vi "1D_Jacobi_eigenvalue_algorithm_v2.vi"() -> ()   [LabVIEW 2020]
uses:
  <vilib>/Analysis/Matrix/Datatypes/RealMatrix.ctl
  <vilib>/Analysis/baseanly.llb/Real A x B.vi
  <vilib>/Analysis/baseanly.llb/Mean (DBL).vi
  <vilib>/Analysis/Matrix/Numeric/Conversions/Array To Matrix - RA2.vi
  <vilib>/Analysis/Matrix/Numeric/Conversions/Matrix To Array - RM.vi
  <vilib>/Analysis/7linalg.llb/Real Eigenvalues and Vectors.vi
  <vilib>/Analysis/Matrix/NI_Matrix.lvlib
  <vilib>/Analysis/NI_AALBase.lvlib
  <vilib>/Analysis/NI_AALPro.lvlib
panel:
  out "New A[k,k]":sgl
  out "[k,k]":i32
  out "after A[k,k]":sgl[][](array[numeric])
  out "before A[k,k]":sgl[][](array[numeric])
  out "Array 3":bool[][](array[boolean])
  out "Numeric":i32
  out "Array 2":i32[](array[numeric])
  out "Array":i32[](array[numeric])
  out "output array":sgl[][](array[numeric])
  out "Real Matrix":T1
  out "percent error":dbl
  out "FPGA Jacobi eigenvalue":sgl[](array[numeric])
  in  "Number of Rotations":i32=100
  out "A":dbl[][](array[numeric])
  out "LabVIEW eigvals":dbl[](array[numeric])
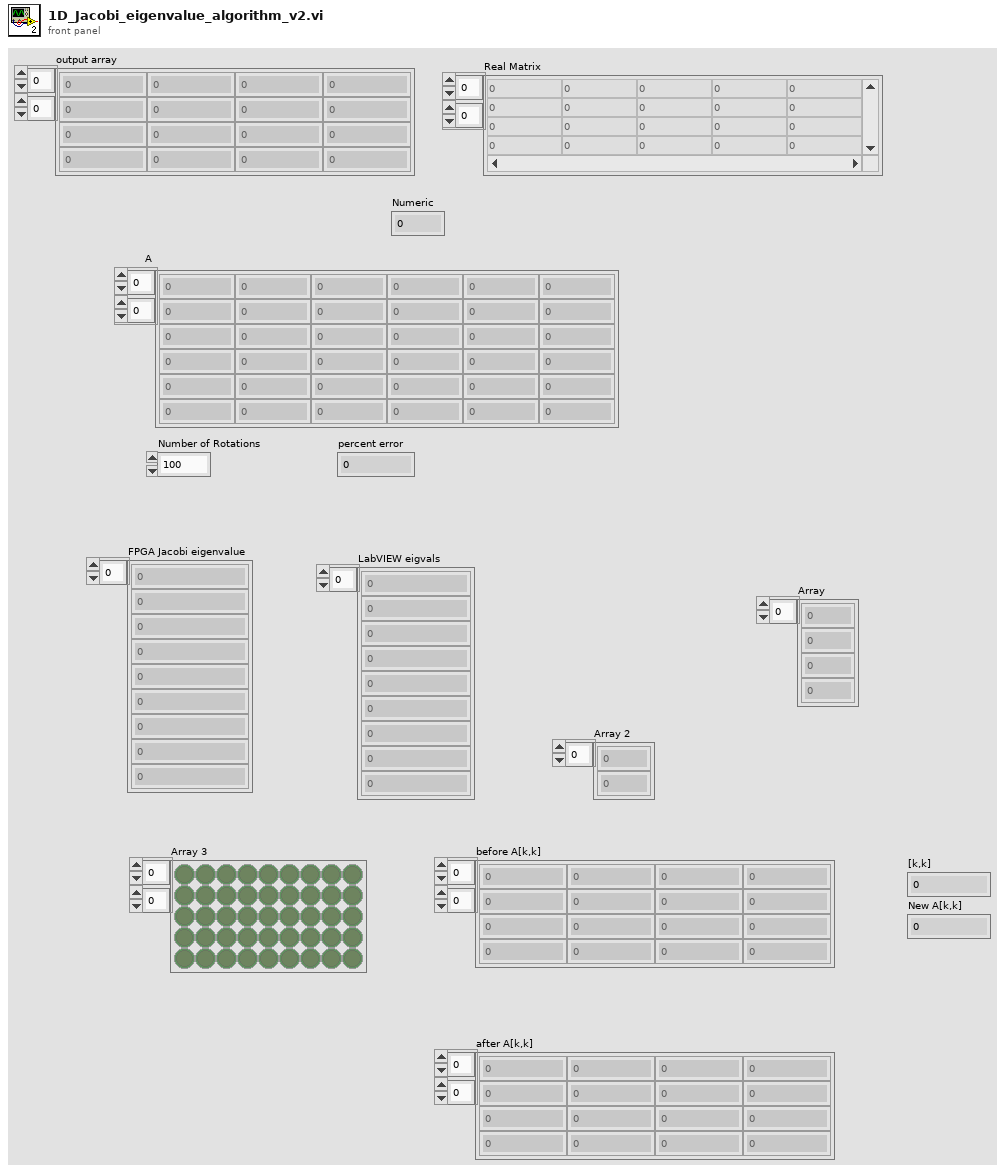
[diagram p1: front panel]
types:
  T1 = typedef "NI_Matrix.lvlib/RealMatrix.ctl" = dbl[][]
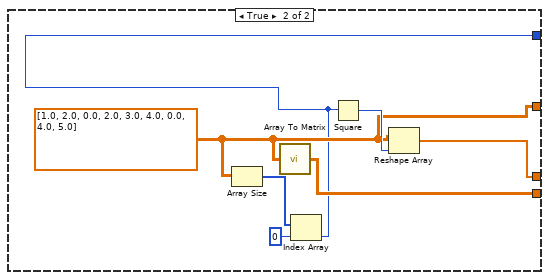
[diagram p2: hidden frame]
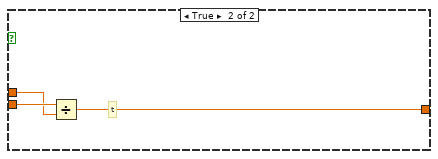
[diagram p4: hidden frame]
diagram:
  n1 = case "Use Troubleshooting Matrix" shown="False" FALSE {
    tunnel: [w13 w32] -> w9
    tunnel: [w14 w31] -> w6
    tunnel: [w12 w29] -> w3
    tunnel: [w11 w26] -> w1
    frame False {
      w11 = 5  # n
      n2 = flat-sequence "Make symmetric matrix" {
        tunnel: [w20] -> w13
        tunnel: [w18] -> w14
        tunnel: [w16] -> w12
        tunnel: w11 -> [w15]
        frame #0 {
          n3 = Multiply(x=w15, y=w15) -> (x*y=w17:i32)
          n4 = for {
            N: w17 -> [_]
            tunnel: [w25] -> w24 mode=indexing
            n5 = Random Number (0-1)() -> (number: 0 to 1=w25:dbl)
          }
          n6 = Reshape Array(w24, w15, w15) -> (w23:dbl[][])
          n7 = call-poly <vilib>:"Array To Matrix.vi"("Real 2D Array"=w23) -> ("Real Matrix"=w22:T1)
          n8 = Transpose Matrix(1:w22) -> (0:w21:T1)
          n9 = call-poly <vilib>:"A x B.vi"("B"=w21, "A"=w22) -> ("A x B"=w20:T1)  [unwired: 1 out]
          n10 = call-poly <vilib>:"Matrix To Array.vi"("Real Matrix"=w20) -> ("Real 2D Array"=w16:dbl[][])
          n11 = Reshape Array(w16, w17) -> (w19:dbl[])
          n12 = To Single Precision Float(number=w19) -> (single precision float=w18:sgl[])
        }
      }
    }
    frame True {
      w29 = sgl[][] [[1.0, 2.0, 0.0], [2.0, 3.0, 4.0], [0.0, 4.0, 5.0]]
      n13 = Array Size(array=w29) -> (size(s)=w28:i32[])
      n14 = call-poly <vilib>:"Array To Matrix.vi"("Real 2D Array"=w29) -> ("Real Matrix"=w32:T1)
      n15 = Index Array(array=w28, index=0) -> (element=w26:i32)
      n16 = Square(x=w26) -> (x^2=w30:i32)
      n17 = Reshape Array(w29, w30) -> (w31:sgl[])
    }
  }
  "A" <- w3
  "Real Matrix" <- w9
  n18 = for "Main Loop: Iterate through each step of the algorithm" {
    N: "Number of Rotations" -> [_]
    tunnel: w1 -> [w71]
    shift-right: [w60] -> w7
    shift-left: w6 -> [w59]
    w35 = 3 ("dimension size")
    w38 = 3 ("dimension size")
    (unwired) 0
    w57 = 3 ("dimension size")
    w74 = sgl 0.0  # A max
    # "i_rotation: 0 to number_of_rotations"
    n19 = Decrement(x=w71) -> (x-1=w73:i32)
    n20 = for "Step #1: Find the location (in k,l) in the top triangle with the greatest value" {
      N: w73 -> [_]
      tunnel: w73 -> [w297]
      shift-right: [w301] -> _
      shift-left: w74 -> [w299]
      tunnel: [w300] -> w68
      tunnel: [w298] -> w72
      tunnel: w59 -> [w296]
      tunnel: w71 -> [w295]
      tunnel: [w293] -> w55 mode=indexing
      tunnel: [w292] -> w54 mode=indexing
      i -> [w293]
      # "i_row loop, 0 to (n-1)"
      n21 = Subtract(x=w297, y=w293) -> (x-y=w302:i32)
      n22 = for "For Loop: j" {
        N: w302 -> [_]
        shift-right: [w311] -> w301
        shift-left: w299 -> [w310]
        tunnel: [w303] -> w300
        tunnel: [w307] -> w298
        tunnel: w296 -> [w320]
        tunnel: w293 -> [w309]
        tunnel: w295 -> [w318]
        tunnel: [w314] -> w294 mode=indexing
        tunnel: [w313] -> w292 mode=indexing
        i -> [w314]
        w304 = 0
        # "j_col, 0 to (n-1-i_row)"
        n23 = Compound Arithmetic op=ADD(w314, w309, 1 ("value")) -> (w306:i32)
        n24 = Multiply(x=w318, y=w309) -> (x*y=w316:i32)
        n25 = Add(x=w316, y=w306) -> (x+y=w315:i32)
        n26 = Index Array(array=w320, index=w315) -> (element=w317:sgl)
        n27 = Absolute Value(x=w317) -> (abs(x)=w312:sgl)
        n28 = Greater Or Equal?(x=w312, y=w310) -> (x >= y?=w313:bool)
        n29 = feedback #1(w304) -> (w308:i32)
        n30 = feedback #2(w304) -> (w305:i32)
        n31 = case "if abs(A[i,j+i+1]) >= A_Max:" shown="False" w313 {
          tunnel: [w323 w326] -> w311
          tunnel: w312 -> [_ w326]
          tunnel: w310 -> [w323 _]
          tunnel: w309 -> [_ w325]
          tunnel: [w322 w325] -> w307
          tunnel: w308 -> [w322 _]
          tunnel: w306 -> [_ w324]
          tunnel: [w321 w324] -> w303
          tunnel: w305 -> [w321 _]
          frame False {
          }
          frame True {
          }
        }
        n32 = feedback-in #1(w307) -> ()
        n33 = feedback-in #2(w303) -> ()
      }
      "Array" <- w294
    }
    "Array 2" <- w55
    "Numeric" <- w72
    "Array 3" <- w54
    n34 = flat-sequence "Step #2: Difference of the orthogonal distance & calculate variables for rotation" {
      tunnel: [w82] -> w67
      tunnel: [w81] -> w66
      tunnel: [w80] -> w65
      tunnel: w72 -> [w86]
      tunnel: w71 -> [w85]
      tunnel: w68 -> [w84]
      tunnel: w59 -> [w83]
      tunnel: [w77] -> w51
      tunnel: [w76] -> w50
      tunnel: [w75] -> w47
      tunnel: [w94] -> w64
      tunnel: w67 -> [w88]
      tunnel: w66 -> [w87]
      tunnel: w65 -> [w89]
      tunnel: [w92] -> w52
      tunnel: w51 -> [w92]
      tunnel: w50 -> [w91]
      tunnel: [w91] -> w49
      tunnel: w47 -> [w90]
      tunnel: [w90] -> w46
      tunnel: [w89] -> w44
      tunnel: [w88] -> w42
      tunnel: [w87] -> w40
      tunnel: w64 -> [w128]
      tunnel: [w128] -> w63
      tunnel: [w127] -> w62
      tunnel: [w126] -> w61
      tunnel: [w125] -> w53
      tunnel: w52 -> [w125]
      tunnel: w49 -> [w124]
      tunnel: [w124] -> w48
      tunnel: w46 -> [w123]
      tunnel: [w123] -> w45
      tunnel: w44 -> [w122]
      tunnel: [w122] -> w43
      tunnel: w42 -> [w121]
      tunnel: [w121] -> w41
      tunnel: w40 -> [w120]
      tunnel: [w120] -> w39
      tunnel: [w149] -> w69
      tunnel: [w150] -> w70
      tunnel: w63 -> [w148]
      tunnel: w62 -> [w150]
      tunnel: w61 -> [w149]
      tunnel: w59 -> [w136]
      tunnel: [w137] -> w58
      tunnel: w53 -> [w143]
      tunnel: w48 -> [w142]
      tunnel: w45 -> [w141]
      tunnel: w43 -> [w140]
      tunnel: w41 -> [w139]
      tunnel: w39 -> [w138]
      tunnel: [w135] -> w36
      tunnel: [w134] -> w33
      frame #0 {
        # "Step #2.1: Get K[I,I], K[k,k], K[k,l]"
        n35 = Multiply(x=w84, y=w85) -> (x*y=w79:i32)
        n36 = Multiply(x=w86, y=w85) -> (x*y=w78:i32)
        n37 = Add(x=w79, y=w84) -> (x+y=w75:i32)
        n38 = Add(x=w78, y=w86) -> (x+y=w76:i32)
        n39 = Add(x=w78, y=w84) -> (x+y=w77:i32)
        n40 = Index Array "A[k,k]"(array=w83, index=w76) -> (element=w81:sgl)
        n41 = Index Array "A[l,l]"(array=w83, index=w75) -> (element=w82:sgl)
        n42 = Index Array "A[k,l]"(array=w83, index=w77) -> (element=w80:sgl)
      }
      frame #1 {
        # "Step #2.2: update t or calculate phi and t, A[k,l] < abs(A_diff)*1e-36"
        n43 = Absolute Value(x=w89) -> (abs(x)=w99:sgl)
        n44 = Subtract(x=w88, y=w87) -> (x-y=w93:sgl)
        n45 = Absolute Value(x=w93) -> (abs(x)=w97:sgl)
        n46 = Multiply(x=w97, y=sgl 1e-36 ("x")) -> (x*y=w98:sgl)
        n47 = Less?(x=w99, y=w98) -> (x < y?=w95:bool)
        n48 = case "A[k,l] < abs(A_diff)*1e-36" shown="False" w95 {
          tunnel: w89 -> [w113 w119]
          tunnel: w93 -> [w110 w118]
          tunnel: [w100 w117] -> w94
          frame False {
            n49 = Multiply(x=w113, y=sgl 2.0) -> (x*y=w111:sgl)
            n50 = Divide(x=w110, y=w111) -> (x/y=w104:sgl)
            n51 = Square(x=w104) -> (x^2=w108:sgl)
            n52 = Increment(x=w108) -> (x+1=w107:sgl)
            n53 = Less?(x=w104, y=sgl 0.0) -> (x < y?=w102:bool)
            n54 = Square Root(x=w107) -> (sqrt(x)=w106:sgl)
            n55 = Absolute Value(x=w104) -> (abs(x)=w109:sgl)
            n56 = Add(x=w106, y=w109) -> (x+y=w105:sgl)
            n57 = Reciprocal(x=w105) -> (1/x=w101:sgl)
            n58 = case shown="True" w102 {
              tunnel: w101 -> [w114 w116]
              tunnel: [w114 w115] -> w100
              frame False {
              }
              frame True {
                n59 = Negate(x=w116) -> (-x=w115:sgl)
              }
            }
          }
          frame True {
            # "t"
            n60 = Divide(x=w119, y=w118) -> (x/y=w117:sgl)
          }
        }
      }
      frame #2 {
        # "Step #2.3: Calculate \"tau\""
        n61 = Square(x=w128) -> (x^2=w131:sgl)
        n62 = Increment(x=w131) -> (x+1=w130:sgl)
        n63 = Square Root(x=w130) -> (sqrt(x)=w129:sgl)
        n64 = Reciprocal(x=w129) -> (1/x=w133:sgl)
        n65 = Multiply(x=w133, y=w128) -> (x*y=w127:sgl)
        n66 = Increment(x=w133) -> (x+1=w132:sgl)
        n67 = Divide(x=w127, y=w132) -> (x/y=w126:sgl)
      }
      frame #3 {
        # "Step #2.4: update the A matrix"
        n68 = Multiply(x=w140, y=w148) -> (x*y=w147:sgl)
        n69 = Subtract(x=w138, y=w147) -> (x-y=w145:sgl)
        "New A[k,k]" <- w145
        n70 = Add(x=w139, y=w147) -> (x+y=w144:sgl)
        n71 = Replace Array Subset "A[k,l]"(array=w136, new element=sgl 0.0 ("y"), index=w143) -> (w135:sgl[])
        n72 = Replace Array Subset "A[k,k]"(array=w135, new element=w145, index=w142) -> (w134:sgl[])
        n73 = Replace Array Subset "A[l,l]"(array=w134, new element=w144, index=w141) -> (w137:sgl[])
        "[k,k]" <- w142
      }
    }
    n74 = Reshape Array(w36, w38, w38) -> (→"before A[k,k]":sgl[][])
    n75 = Reshape Array(w33, w35, w35) -> (→"after A[k,k]":sgl[][])
    n76 = Reshape Array(w58, w57, w57) -> (→"output array":sgl[][])
    n77 = flat-sequence "Step #3: Rotate around the high value point" {
      tunnel: w72 -> [w156]
      tunnel: w58 -> [w165]
      tunnel: w71 -> [w157]
      tunnel: w70 -> [w151]
      tunnel: w69 -> [w152]
      tunnel: w68 -> [w155]
      tunnel: [w154] -> w60
      frame #0 {
        n78 = for {
          N: w156 -> [_]
          tunnel: w157 -> [w266]
          tunnel: w156 -> [w265]
          tunnel: w151 -> [w260]
          tunnel: w152 -> [w264]
          tunnel: w155 -> [w261]
          shift-right: [w252] -> w164
          shift-left: w165 -> [w259]
          i -> [w267]
          # "i loop, 0 to k"
          n79 = Multiply(x=w266, y=w267) -> (x*y=w262:i32)
          n80 = Add(x=w262, y=w261) -> (x+y=w263:i32)
          n81 = Add(x=w262, y=w265) -> (x+y=w258:i32)
          n82 = flat-sequence "Step 3.1: Update A" {
            tunnel: w264 -> [w270]
            tunnel: w263 -> [w271]
            tunnel: w260 -> [w268]
            tunnel: w259 -> [w274]
            tunnel: w258 -> [w269]
            tunnel: [w272] -> w257
            tunnel: [w271] -> w256
            tunnel: [w270] -> w255
            tunnel: [w269] -> w254
            tunnel: [w268] -> w253
            tunnel: w257 -> [w291]
            tunnel: w256 -> [w281]
            tunnel: w255 -> [w290]
            tunnel: w254 -> [w287]
            tunnel: w253 -> [w285]
            tunnel: [w280] -> w252
            frame #0 {
              # "Step 3.1.1: Update A[i,k]"
              n83 = Index Array "A[i,l]"(array=w274, index=w271) -> (element=w277:sgl)
              n84 = Index Array "A[i,k]"(array=w274, index=w269) -> (element=w279:sgl)
              n85 = Multiply(x=w279, y=w270) -> (x*y=w278:sgl)
              n86 = Add(x=w277, y=w278) -> (x+y=w276:sgl)
              n87 = Multiply(x=w276, y=w268) -> (x*y=w275:sgl)
              n88 = Subtract(x=w279, y=w275) -> (x-y=w273:sgl)
              n89 = Replace Array Subset "A[i,k]"(array=w274, new element=w273, index=w269) -> (w272:sgl[])
            }
            frame #1 {
              # "# Step 3.1.2: Update A[i,l]"
              n90 = Index Array "A[i,k]"(array=w291, index=w287) -> (element=w289:sgl)
              n91 = Index Array "A[i,l]"(array=w291, index=w281) -> (element=w283:sgl)
              n92 = Multiply(x=w283, y=w290) -> (x*y=w288:sgl)
              n93 = Subtract(x=w289, y=w288) -> (x-y=w286:sgl)
              n94 = Multiply(x=w286, y=w285) -> (x*y=w284:sgl)
              n95 = Add(x=w283, y=w284) -> (x+y=w282:sgl)
              n96 = Replace Array Subset "A[i,l]"(array=w291, new element=w282, index=w281) -> (w280:sgl[])
            }
          }
        }
        n97 = Subtract(x=w155, y=1) -> (x-y=w163:i32)
        n98 = Subtract(x=w163, y=w156) -> (x-y=w161:i32)
        n99 = for {
          N: w161 -> [_]
          shift-right: [w227] -> w153
          shift-left: w164 -> [w225]
          tunnel: w156 -> [w223]
          tunnel: w157 -> [w219]
          tunnel: w155 -> [w217]
          tunnel: w152 -> [w215]
          tunnel: w151 -> [w213]
          i -> [w222]
          # "i loop, 0 to (l-1-k)"
          n100 = Multiply(x=w223, y=w219) -> (x*y=w221:i32)
          n101 = Compound Arithmetic op=ADD(w222, 1 ("value"), w223) -> (w220:i32)
          n102 = Add(x=w221, y=w220) -> (x+y=w216:i32)
          n103 = Multiply(x=w220, y=w219) -> (x*y=w218:i32)
          n104 = Add(x=w218, y=w217) -> (x+y=w214:i32)
          n105 = flat-sequence "Step 3.2: Update A" {
            tunnel: [w239] -> w226
            tunnel: w225 -> [w238]
            tunnel: w216 -> [w229]
            tunnel: w215 -> [w230]
            tunnel: w214 -> [w231]
            tunnel: w213 -> [w228]
            tunnel: [w231] -> w212
            tunnel: [w230] -> w211
            tunnel: [w229] -> w210
            tunnel: [w228] -> w209
            tunnel: [w251] -> w227
            tunnel: w226 -> [w248]
            tunnel: w212 -> [w250]
            tunnel: w211 -> [w249]
            tunnel: w210 -> [w247]
            tunnel: w209 -> [w243]
            frame #0 {
              # "Step 3.2.1: Update A[k,i+1+k?]"
              n106 = Index Array "A[k,i+1+k?]"(array=w238, index=w229) -> (element=w234:sgl)
              n107 = Index Array "A[i+1+k,l?]"(array=w238, index=w231) -> (element=w237:sgl)
              n108 = Multiply(x=w234, y=w230) -> (x*y=w236:sgl)
              n109 = Add(x=w237, y=w236) -> (x+y=w235:sgl)
              n110 = Multiply(x=w235, y=w228) -> (x*y=w233:sgl)
              n111 = Subtract(x=w234, y=w233) -> (x-y=w232:sgl)
              n112 = Replace Array Subset "A[k,i+1+k?]"(array=w238, new element=w232, index=w229) -> (w239:sgl[])
            }
            frame #1 {
              # "Step 3.2.2: Update A[i+1+k,l?]"
              n113 = Index Array "A[i+1+k,l?]"(array=w248, index=w250) -> (element=w241:sgl)
              n114 = Multiply(x=w241, y=w249) -> (x*y=w245:sgl)
              n115 = Index Array "A[k,i+1+k?]"(array=w248, index=w247) -> (element=w246:sgl)
              n116 = Subtract(x=w246, y=w245) -> (x-y=w244:sgl)
              n117 = Multiply(x=w244, y=w243) -> (x*y=w242:sgl)
              n118 = Add(x=w241, y=w242) -> (x+y=w240:sgl)
              n119 = Replace Array Subset "A[i+1+k,l?]"(array=w248, new element=w240, index=w250) -> (w251:sgl[])
            }
          }
        }
        n120 = Subtract(x=w157, y=1) -> (x-y=w159:i32)
        n121 = Subtract(x=w159, y=w155) -> (x-y=w158:i32)
        n122 = for {
          N: w158 -> [_]
          tunnel: w157 -> [w180]
          tunnel: w156 -> [w184]
          tunnel: w155 -> [w179]
          shift-right: [w176] -> w154
          shift-left: w153 -> [w174]
          tunnel: w152 -> [w172]
          tunnel: w151 -> [w170]
          i -> [w183]
          # "i loop, 0 to (n-1-l)"
          n123 = Multiply(x=w180, y=w179) -> (x*y=w178:i32)
          n124 = Multiply(x=w184, y=w180) -> (x*y=w181:i32)
          n125 = Compound Arithmetic op=ADD(w183, 1 ("value"), w179) -> (w177:i32)
          n126 = Add(x=w178, y=w177) -> (x+y=w171:i32)
          n127 = Add(x=w181, y=w177) -> (x+y=w173:i32)
          n128 = flat-sequence "Step 3.3: Update A" {
            tunnel: [w190] -> w175
            tunnel: w174 -> [w191]
            tunnel: w173 -> [w186]
            tunnel: w172 -> [w187]
            tunnel: w171 -> [w188]
            tunnel: w170 -> [w185]
            tunnel: [w188] -> w169
            tunnel: [w187] -> w168
            tunnel: [w186] -> w167
            tunnel: [w185] -> w166
            tunnel: [w208] -> w176
            tunnel: w175 -> [w205]
            tunnel: w169 -> [w207]
            tunnel: w168 -> [w206]
            tunnel: w167 -> [w204]
            tunnel: w166 -> [w200]
            frame #0 {
              # "Step 3.3.1: Update A[k,i+1+l?]"
              n129 = Index Array "A[k,i+1+l?]"(array=w191, index=w186) -> (element=w193:sgl)
              n130 = Multiply(x=w193, y=w187) -> (x*y=w196:sgl)
              n131 = Index Array "A[l,i+1+l?]"(array=w191, index=w188) -> (element=w195:sgl)
              n132 = Add(x=w196, y=w195) -> (x+y=w194:sgl)
              n133 = Multiply(x=w194, y=w185) -> (x*y=w192:sgl)
              n134 = Subtract(x=w193, y=w192) -> (x-y=w189:sgl)
              n135 = Replace Array Subset "A[i+1+k,l?]"(array=w191, new element=w189, index=w186) -> (w190:sgl[])
            }
            frame #1 {
              # "Step 3.3.2: Update A[l,i+1+l?]"
              n136 = Index Array "A[l,i+1+l?]"(array=w205, index=w207) -> (element=w198:sgl)
              n137 = Multiply(x=w198, y=w206) -> (x*y=w202:sgl)
              n138 = Index Array "A[k,i+1+l?]"(array=w205, index=w204) -> (element=w203:sgl)
              n139 = Subtract(x=w203, y=w202) -> (x-y=w201:sgl)
              n140 = Multiply(x=w201, y=w200) -> (x*y=w199:sgl)
              n141 = Add(x=w199, y=w198) -> (x+y=w197:sgl)
              n142 = Replace Array Subset "A[l,i_1+l?]"(array=w205, new element=w197, index=w207) -> (w208:sgl[])
            }
          }
        }
      }
    }
  }
  n143 = call-poly <vilib>:"Eigenvalues and Vectors.vi"("Input Matrix"=w9) -> ("Eigenvalues"=w10:cdb[])  [unwired: 2 in, 2 out]
  n144 = Complex To Re/Im(x + iy=w10) -> (x=w4:dbl[])  [unwired: 1 out]
  n145 = flat-sequence "Step 4: extract the Eigen values from the diagonal" {
    tunnel: w7 -> [w329]
    tunnel: w1 -> [w328]
    tunnel: [w327] -> w5
    frame #0 {
      n146 = for "Eigenvalue vector" {
        N: w328 -> [_]
        tunnel: [sgl 0.0] -> w330 mode=indexing
      }
      n147 = for "Eigenvalue vector" {
        N: w328 -> [_]
        shift-right: [w337] -> w327
        shift-left: w330 -> [w338]
        tunnel: w329 -> [w336]
        tunnel: w328 -> [w335]
        i -> [w333]
        n148 = Multiply(x=w335, y=w333) -> (x*y=w334:i32)
        n149 = Add(x=w334, y=w333) -> (x+y=w332:i32)
        n150 = Index Array "A[k,i+1+l?]"(array=w336, index=w332) -> (element=w331:sgl)
        n151 = Replace Array Subset(array=w338, new element=w331, index=w333) -> (w337:sgl[])
      }
    }
  }
  n152 = flat-sequence "Calculate the percent error" {
    tunnel: w5 -> [w351]
    tunnel: w4 -> [w350]
    frame #0 {
      n153 = Sort 1D Array(array=w350) -> (sorted array=w349:dbl[])
      "LabVIEW eigvals" <- w349
      n154 = Sort 1D Array(array=w351) -> (sorted array=w348:sgl[])
      "FPGA Jacobi eigenvalue" <- w348
      n155 = To Single Precision Float(number=w349) -> (single precision float=w345:sgl[])
      n156 = Subtract(x=w348, y=w345) -> (x-y=w347:sgl[])
      n157 = Absolute Value(x=w347) -> (abs(x)=w346:sgl[])
      n158 = Divide(x=w346, y=w345) -> (x/y=w344:sgl[])
      n159 = Absolute Value(x=w344) -> (abs(x)=w343:sgl[])
      n160 = call-poly <vilib>:"Mean.vi"("X"=w343) -> ("mean"=w342:dbl)  [unwired: 1 out]
      n161 = Multiply(x=w342, y=100.0) -> (x*y=→"percent error":dbl)
    }
  }
